vi "onTestSlippage.vi"(7 "DefineTest in":refnum<class "DefineTest.lvclass">, 11 "Leaf.TestCase":refnum<class "Leaf.TestCase.lvclass">) -> (0 "error out":errorcluster, 3 "Leaf.TestCase":refnum<class "Leaf.TestCase.lvclass">)   [LabVIEW 2021, in "Bananas.lvlib" / "DefineTest.lvclass"]
uses:
  DefineTest.lvclass
  DefineTest.lvclass/DefineTest.ctl
  Leaf.TestCase/Leaf.TestCase.lvclass
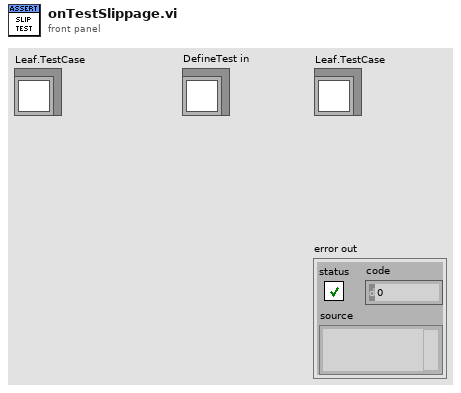
[diagram p1: front panel]
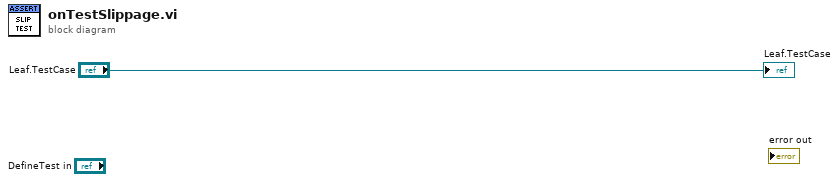
[diagram p0: block diagram]
diagram:
  "Leaf.TestCase" <- "Leaf.TestCase"
